vi "Constants.vi"() -> ()   [LabVIEW 2023, in "J1939 Addon Shared.lvlib"]
uses:
  J1939 Addon Shared.lvlib
panel:
  in  "Node.ForceSA":string="Node.ForceSA"
  in  "Refs.Override":string="OverrideSignals"
  in  "Protected Channel GUID":string="F82EDF65-1315-4943-9C5D-FF4C2375D45C"
  in  "Help.FileName":string="J1939 Addon.chm"
  in  "Refs.CountersAndProtections":string="CountersAndProtections"
  in  "Refs.CounterAndProtectionSignals":string="CounterAndProtectionSignals"
  in  "Protection Value GUID":string="fe15317e-b165-43a3-9d5b-faa422f66725"
  in  "Counter Value GUID":string="4a3d9735-5760-4a43-a9a4-de30f92d91fe"
  in  "Signal Out Page GUID":string="7ef80e0d-db85-46b1-8781-0be83a57b682"
  in  "Outgoing Cyclic Event Name":string="Cyclic Event"
  in  "Outgoing Cyclic Event Page GUID":string="88701071-4de5-4e42-926f-383c42931fd6"
  in  "Node.IncludeDA":string="Node.IncludeDA"
  in  "Outgoing Frame Page GUID":string="032E9F13-B321-4033-8075-157E9AAD2CDE"
  in  "SPN.ScaleOff":string="SPN.ScaleOff"
  in  "SPN.ScaleFac":string="SPN.ScaleFac"
  in  "SPN.Bytes":string="SPN.Bytes"
  in  "Node.Address":string="Node.Address"
  in  "Node.Name":string="Node.Name"
  in  "XNET.Outgoing.Decimation":string="XNET.Outgoing.Decimation"
  in  "XNET.Incoming.Decimation":string="XNET.Incoming.Decimation"
  in  "XNET.Termination":string="XNET.Termination"
  in  "XNET.Rate":string="XNET.Rate"
  in  "XNET.Port":string="XNET.Port"
  in  "XNET.Cluster":string="XNET.Cluster"
  in  "XNET.Database":string="XNET.Database"
  in  "Frame.Disable Transmission":string="Disable Transmission"
  in  "Frame.Transmit Trigger":string="Transmit Trigger"
  in  "Frame.Trigger":string="Frame.Trigger"
  in  "Frame.Disable":string="Frame.Disable"
  in  "Time Difference GUID":string="a95322d4-6192-45f9-b3fd-7ebfccdab5eb"
  in  "Time Difference Name":string="Time Difference"
  in  "Receive Time Name":string="Receive Time"
  in  "Information Name":string="Frame Information"
  in  "Receive Time GUID":string="848e2b92-ac0f-419e-baf3-639235006264"
  in  "Information Page GUID":string="ad57ac2e-75ac-4620-acbf-127be53549ac"
  in  "Outgoing Cyclic Name":string="Cyclic"
  in  "Outgoing Cyclic GUID":string="edd83735-91d2-4d0c-b78a-b1a4a8adab0a"
  in  "Refs.InternalResp":string="InternalResp"
  in  "Refs.InternalCmd":string="InternalCmd"
  in  "Protect Lamp":string="Protect Lamp"
  in  "Amber Warning":string="Amber Warning"
  in  "Red Stop":string="Red Stop"
  in  "Malfunction Indicator":string="Malfunction Indicator"
  in  "Enable?":string="Enable"
  in  "SPN":string="SPN"
  in  "Occurrance":string="Occurrance"
  in  "FMI":string="FMI"
  in  "Simulation Page Name":string="Simulate"
  in  "Monitor Tool Page Name":string="Monitor"
  in  "DM2 Page Name":string="DM2 Previous DTCs"
  in  "DTC Page Name":string="DTC"
  in  "Simulated Diagnostics Page Name":string="Diagnostics"
  in  "Sim Device Page Name":string="Device"
  in  "DM1 Page Name":string="DM1 Active DTCs"
  in  "Simulation GUID":string="5d542ba3-f934-47c8-8526-922e6671f75c"
  in  "Monitor Tool GUID":string="ff8806fd-5187-43dd-8ad2-27d2e390b985"
  in  "DM2 GUID":string="a6e56184-1e6e-4172-a68a-86fd02f8cb1d"
  in  "DTC GUID":string="3533116e-8365-4b51-8f4f-44b0c5dae14b"
  in  "Simulated Diagnostics GUID":string="ab47f5e2-17b5-4786-91a9-aa1b83ce3202"
  in  "Sim Device GUID":string="a71bef71-deb0-46ee-be35-fd124c3f2929"
  in  "DM1 GUID":string="c2782be08-a048-47b9-a94e-6f4691487fca"
  in  "J1939 Compiled Settings":string="J1939 Compiled Settings"
  in  "RT Bitfile Location":path=path "c:/ni-rt/NIVeriStand/XNET"
  in  "RIO Device 986x":string="RIO Device 986x"
  in  "Enable 986x":string="Enable 986x"
  in  "Bitfile 986x":string="Bitfile 986x"
  in  "Diagnostic Channel GUID":string="b62ef38f-3fa0-48a7-a2a3-2fe65e89e411"
  in  "DTC Clear Type":string="DTC Clear Type"
  in  "Requested DTC Status":string="Requested DTC Status"
  in  "# of DTCs Found":string="# of DTCs Found"
  in  "Address to Query":string="Address to Query"
  in  "Expected DTC":string="Expected DTC"
  in  "Diagnostic Command Status":string="Diagnostic Command Status"
  in  "Diagnostic Error Code":string="Diagnostic Error Code"
  in  "Diagnostic Command":string="Diagnostic Command"
  in  "Clear DTCs Page Name":string="Clear DTCs"
  in  "Clear DTCs GUID":string="5fe7a49a-076c-4c99-b5c3-65c554d9b468"
  in  "Verify DTCs Page Name":string="Verify DTC"
  in  "Verify DTCs GUID":string="a36e014a-9629-4cf0-b875-c21cd502bc82"
  in  "Diagnostics Page Name":string="Diagnostics"
  in  "Diagnostics GUID":string="fc9df2d5-46c1-45d0-98f7-1a68aab098d6"
  in  "Main Page GUID Disabled":string="A9661AD5-DF74-BF37-4CA8-5E0EF738F6FD"
  in  "Trigger Request":string="Trigger Request"
  in  "Request Destination":string="Request Destination"
  in  "Request PGN":string="Request PGN"
  in  "Request Section Name":string="Requests"
  in  "Debug Enable Name":string="Debug Enable"
  in  "Status Section Name":string="Status"
  in  "Frame.ID":string="ID"
  in  "Outgoing Event Page Name":string="Event Triggered"
  in  "Outgoing Page Name":string="Outgoing"
  in  "Incoming Single Point Page Name":string="Single Point"
  in  "Incoming Page Name":string="Incoming"
  in  "Incoming Frame Page GUID":string="AA452EA6-A39D-713C-6D0F-1CFCE5C8BC25"
  in  "Signal Page GUID":string="FC3154D4-9B07-90D1-2A8F-6657A6DF127D"
  in  "Outgoing Event Page GUID":string="66CA57DF-0030-7FEB-7718-A68954D700B8"
  in  "Outgoing Page GUID":string="AF90FC7A-ACD0-CE24-9513-B991C453EC9C"
  in  "Incoming Single Point Page GUID":string="F09FE425-7E71-8634-77FE-097EFBD4E192"
  in  "Incoming Page GUID":string="AD3E1237-0B33-86CD-C074-2ECB9FA086C8"
  in  "Main Page GUID":string="5D441869-002F-93F2-B7E0-78053FA04717"
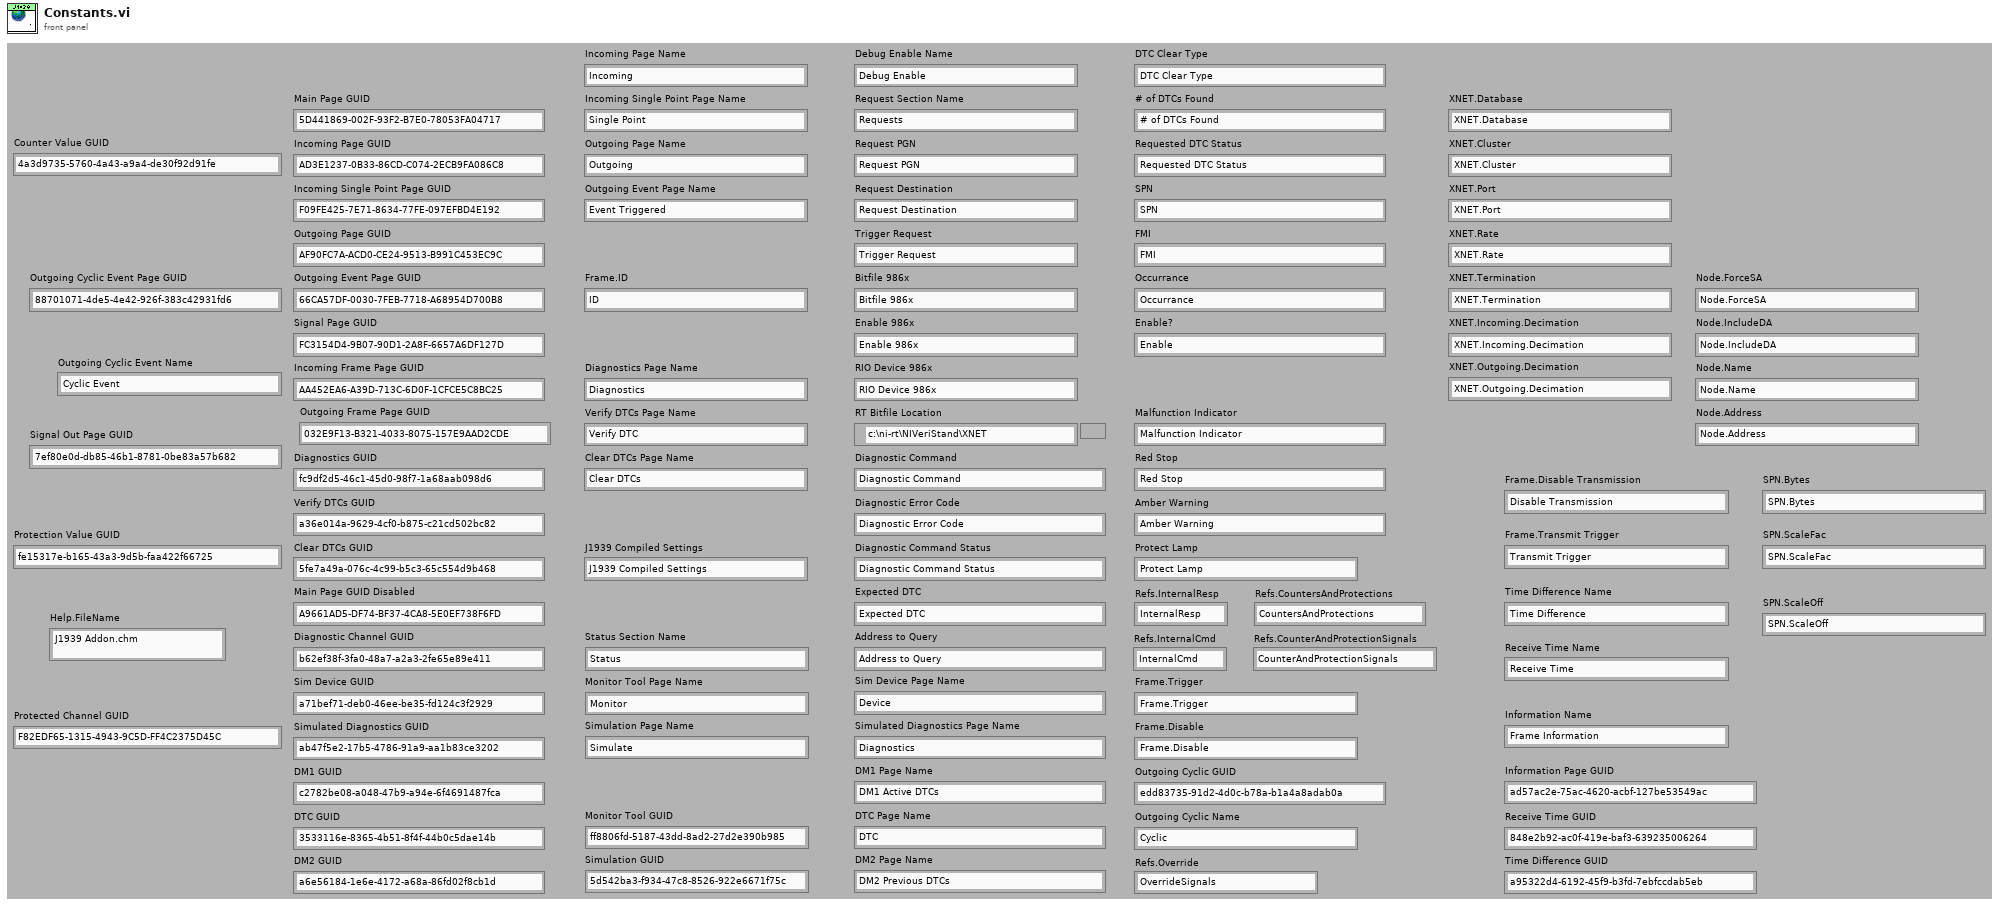
[diagram p1: front panel]
diagram:
